vi "dbsys_status.vi"() -> (0 "Статус":string)   [LabVIEW 2017]
uses:
  D:/DBSys/VI/DBSysCore.dll
  DBSysCore.dll
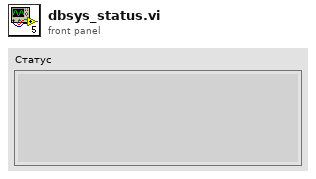
[diagram p1: front panel]
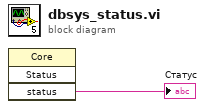
[diagram p0: block diagram]
diagram:
  n1 = invoke class="Core" method="Status"() -> ("status"=→"Статус":string)  [unwired: 4 in, 3 out]
